vi "Refname to String (Joystick).vi"(1 "Joystick Refname":T1) -> (0 "Refnum Name":string)   [LabVIEW 2014]
uses:
  Refname Enum (Joystick).ctl
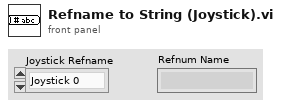
[diagram p1: front panel]
types:
  T1 = typedef "Refname Enum (Joystick).ctl" = enum16{"Joystick 0", "Joystick 1", "Joystick 2", "Joystick 3"}
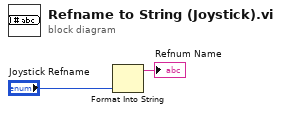
[diagram p0: block diagram]
diagram:
  n1 = Format Into String("Joystick Refname") -> (resulting string=→"Refnum Name":string)  [unwired: 3 in, 1 out]
